vi "Check Start.vi"(8 "error in (no error)":errorcluster, 11 "TCP Comm":T1) -> (0 "error out":errorcluster, 3 "Start":bool)   [LabVIEW 2020, in "TinyTCP.lvlib"]
uses:
  TinyTCP.lvlib
  Instance.ctl
  Ref Data.ctl
  State.ctl
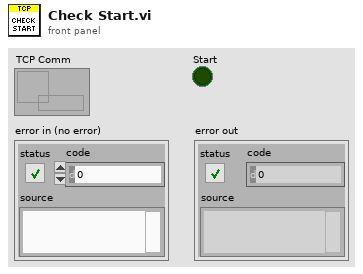
[diagram p1: front panel]
types:
  T1 = typedef "TinyTCP.lvlib/Instance.ctl" = refnum<data-value>
  T2 = typedef "TinyTCP.lvlib/State.ctl" = enum16{"Idle", "Starting", "Connecting", "Connected", "Disconnecting", "Stopped"}
  T3 = typedef "TinyTCP.lvlib/Ref Data.ctl" = cluster{"TCP":refnum<k5>, "State":T2, "Server":bool, "Host":string, "Port":u16, "Listener":refnum<k5>, "Start":bool, "Disconnect":bool, "TCP Valid":bool, "TLS Enabled":bool, "Immutable TLS":refnum<k36>, "Certificate DN":string, "local-port":u16}
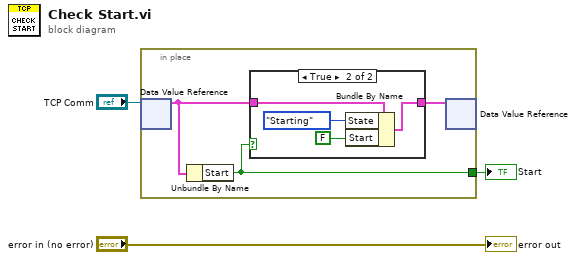
[diagram p0: block diagram]
diagram:
  n1 = in-place {
    in-place-border: [w4] -> w1
    n2 = in-place-dvr #1("TCP Comm") -> (w6:T3)  [unwired: 1 out]
    n3 = Unbundle By Name(w6) -> ("Start"=w4:bool)
    n4 = case shown="True" w4 {
      tunnel: w6 -> [w7 w11]
      tunnel: [w7 w8] -> w5
      frame False {
      }
      frame True {
        n5 = Bundle By Name(cluster=w11, "State"=State."Starting", "Start"=FALSE) -> (w8:T3)
      }
    }
    n6 = in-place-dvr #1(w5) -> ()  [unwired: 2 out]
  }
  "Start" <- w1
  "error out" <- "error in (no error)"
